vi "read_attributes.vi"(8 "error in (no error)":errorcluster, 11 "KernelPCA in":refnum<class "KernelPCA.lvclass">) -> (0 "error out":errorcluster, 2 "attributes":T1, 3 "KernelPCA out":refnum<class "KernelPCA.lvclass">)   [LabVIEW 2020, in "KernelPCA.lvclass"]
uses:
  KernelPCA.lvclass
  Controls/kernel_pca_attributes.ctl
  KernelPCA.lvclass/KernelPCA.ctl
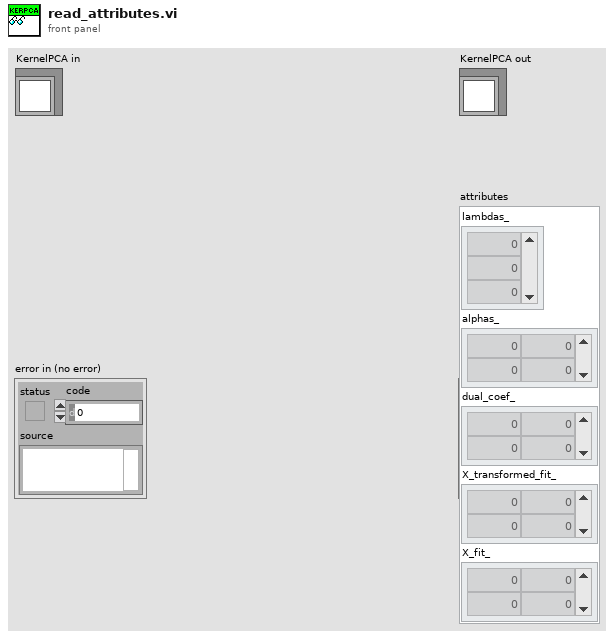
[diagram p1: front panel]
types:
  T1 = typedef "kernel_pca_attributes.ctl" = cluster{"lambdas_":dbl[], "alphas_":dbl[][], "dual_coef_":dbl[][], "X_transformed_fit_":dbl[][], "X_fit_":dbl[][]}
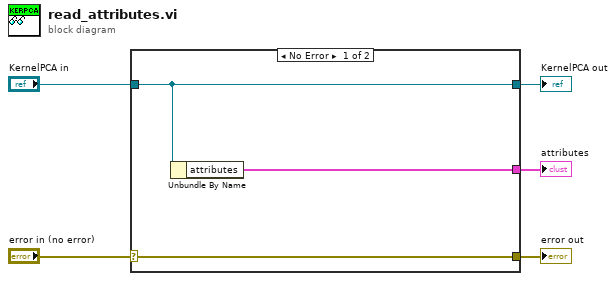
[diagram p0: block diagram]
diagram:
  n1 = case shown="No Error" "error in (no error)" {
    selector: "error in (no error)" -> [w8 w9]
    tunnel: [w8 w9] -> w4
    tunnel: [w7 w10] -> w2
    tunnel: "KernelPCA in" -> [w7 w10]
    tunnel: [w6 _] -> w1
    frame No Error {
      n2 = Unbundle By Name(w7) -> ("attributes"=w6:T1)
    }
    frame Error {
    }
  }
  "error out" <- w4
  "KernelPCA out" <- w2
  "attributes" <- w1
